vi "SuperAuto.vi"() -> ()   [LabVIEW 2014]
uses:
  Support Files/SuperAutoStates.ctl
  Support Files/Global Data!!!.vi
  <vilib>/addons/control/pid/pid.llb/PID (DBL).vi
  <vilib>/addons/control/pid/NI_PID_pid.lvlib
panel:
  in  "liftEnc":dbl
  in  "elevator":dbl
  in  "autoLift":bool
  in  "rightEnc":dbl
  in  "leftEnc":dbl
  in  "manual?":bool
  in  "ElevatorStateMachine":bool
  in  "gyroAngle":dbl
  in  "Turn":dbl
  in  "Power":dbl
  in  "Extend":bool
  in  "SecondStage":bool
  in  "FirstStage":bool
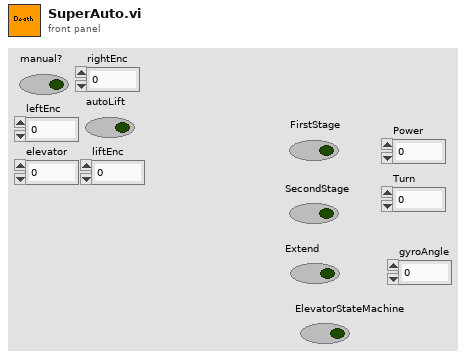
[diagram p1: front panel]
types:
  T1 = typedef "SuperAutoStates.ctl" = enum16{"Grasp RC", "Turn", "Release", "Retract", "2-Stage Process", "Straigten", "Drive Forward", "Done"}
  T2 = cluster{"proportional gain (Kc)":dbl, "integral time (Ti, min)":dbl, "derivative time (Td, min)":dbl}
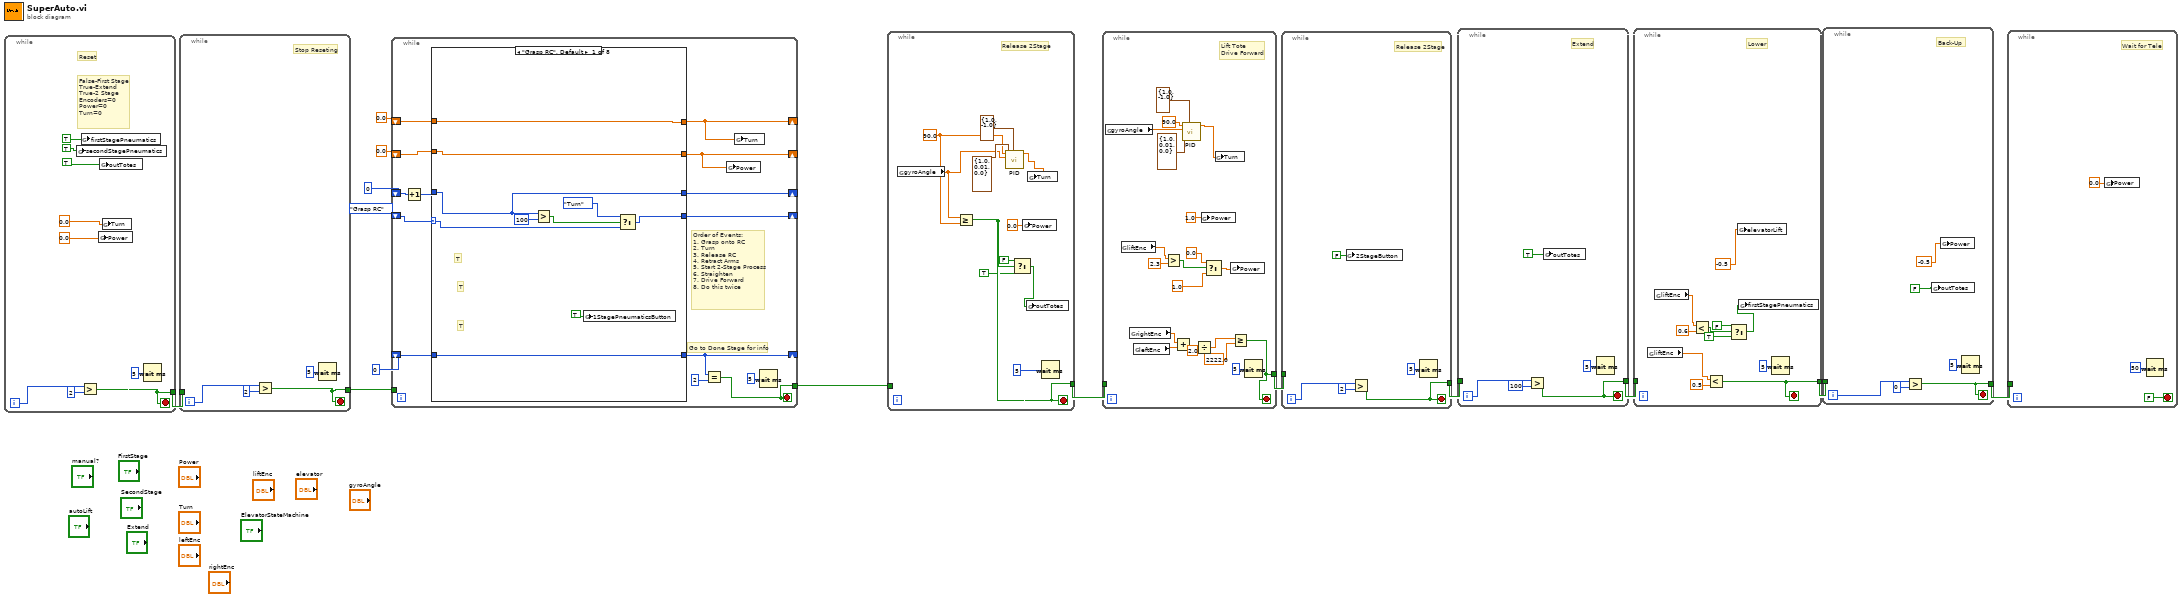
[diagram p0: block diagram]
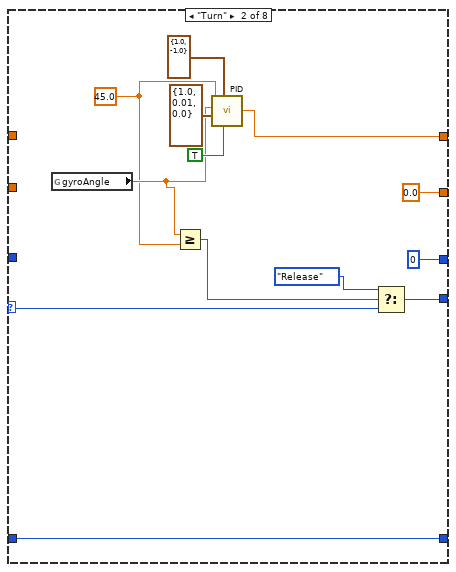
[diagram p2: hidden frame]
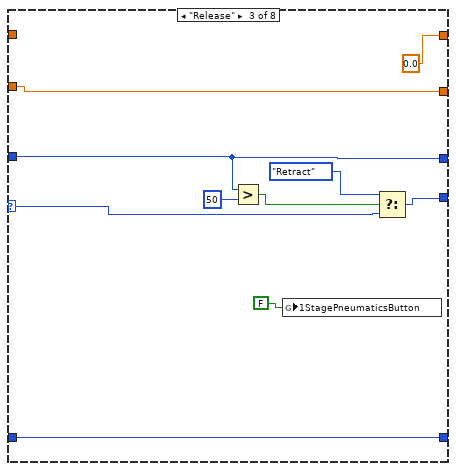
[diagram p3: hidden frame]
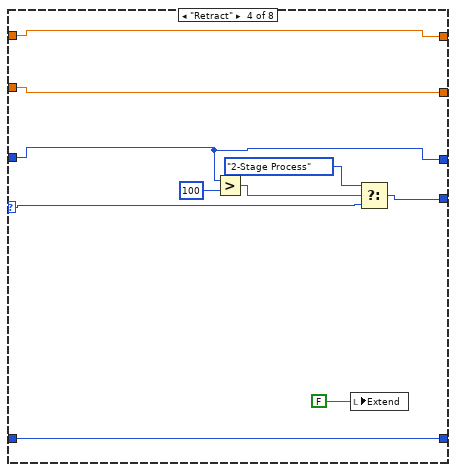
[diagram p4: hidden frame]
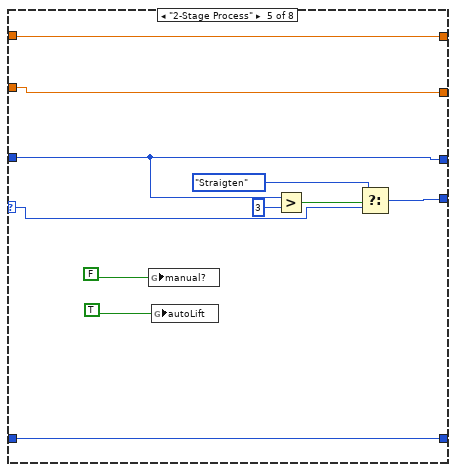
[diagram p5: hidden frame]
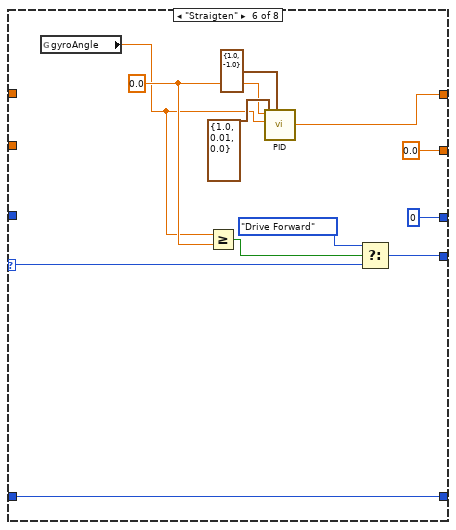
[diagram p6: hidden frame]
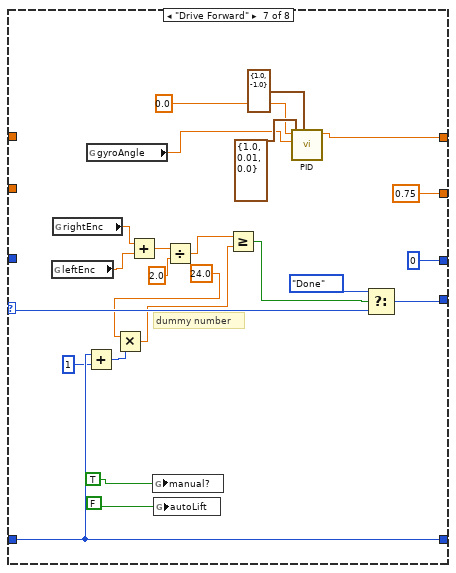
[diagram p7: hidden frame]
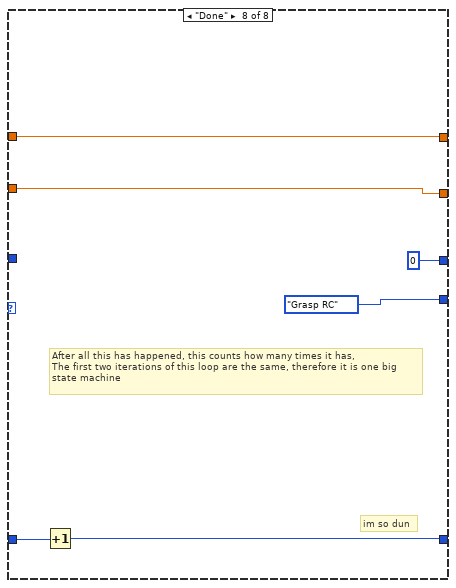
[diagram p8: hidden frame]
diagram:
  n1 = while {
    tunnel: [w20] -> w14
    i -> [w23]
    stop <- w20 stop-if-true
    # "False-First Stage\nTrue-Extend\nTrue-2 Stage\nEncoders=0\nPower=0\nTurn=0"
    # "Reset"
    n2 = global write "Global Data!!!.vi" "secondStagePneumatics"(TRUE) -> ()
    n3 = global write "Global Data!!!.vi" "firstStagePneumatics"(TRUE) -> ()
    n4 = Greater?(x=w23, y=2) -> (0:w20:bool)
    n5 = global write "Global Data!!!.vi" "Power"(0.0) -> ()
    n6 = global write "Global Data!!!.vi" "outTotes"(TRUE) -> ()
    n7 = global write "Global Data!!!.vi" "Turn"(0.0) -> ()
    n8 = Wait (ms)(milliseconds to wait=u32 5) -> ()  [unwired: 1 out]
  }
  n9 = while {
    tunnel: w14 -> [_]
    tunnel: [w24] -> w11
    i -> [w27]
    stop <- w24 stop-if-true
    # "Stop Reseting"
    n10 = Greater?(x=w27, y=2) -> (0:w24:bool)
    n11 = Wait (ms)(milliseconds to wait=u32 5) -> ()  [unwired: 1 out]
  }
  n12 = while {
    shift-right: [w40] -> _
    shift-left: SuperAutoStates."Grasp RC" -> [w41]
    shift-right: [w36] -> _
    shift-left: u32 0 ("milliseconds to wait") -> [w38]
    shift-right: [w29] -> _
    shift-left: 0.0 ("output") -> [w34]
    shift-right: [w28] -> _
    shift-left: 0.0 -> [w35]
    tunnel: w11 -> [_]
    shift-right: [w32] -> _
    shift-left: u32 0 ("milliseconds to wait") -> [w33]
    tunnel: [w30] -> w4
    stop <- w30 stop-if-true
    # "Go to Done Stage for info"
    # "Order of Events: \n1. Grasp onto RC\n2. Turn\n3. Release RC\n4. Retract Arms\n5. Start 2-Stage Process\n6. Straighten\n7. Drive Forward\n8. Do this twice"
    n13 = Increment(x=w38) -> (x+1=w37:u32)
    n14 = case shown="\"Grasp RC\", Default" w41 {
      selector: w41 -> [w51 w62 w69 w77 w92 w102 w126 _]
      tunnel: [w45 w55 0.0 ("output") w82 w89 w99 w120 w133] -> w29
      tunnel: [w44 0.0 w68 w81 w88 0.0 0.75 w132] -> w28
      tunnel: [w50 w63 w66 w75 w94 w103 w127 SuperAutoStates."Grasp RC"] -> w40
      tunnel: w37 -> [w46 _ w70 w76 w87 _ _ _]
      tunnel: [w46 u32 0 w70 w76 w87 u32 0 u32 0 u32 0] -> w36
      tunnel: w35 -> [w44 _ w68 w81 w88 _ _ w132]
      tunnel: w34 -> [w45 _ _ w82 w89 _ _ w133]
      tunnel: [w43 w58 w67 w84 w95 w107 w115 w135] -> w32
      tunnel: w33 -> [w43 w58 w67 w84 w95 w107 w115 w136]
      frame "Grasp RC", Default {
        # "T"
        # "T"
        # "T"
        n15 = Greater?(x=w46, y=u32 100) -> (0:w48:bool)
        n16 = global write "Global Data!!!.vi" "1StagePneumaticsButton"(TRUE) -> ()
        n17 = Select(t=SuperAutoStates."Turn", s=w48, f=w51) -> (s? t:f=w50:T1)
      }
      frame "Turn" {
        w52 = 45.0 ("setpoint")
        n18 = global read "Global Data!!!.vi" "gyroAngle"() -> (w53:dbl)
        n19 = Greater Or Equal?(x=w53, y=w52) -> (x >= y?=w60:bool)
        n20 = call-poly <vilib>:"PID.vi"("reinitialize? (F)"=TRUE, "output range"=cluster{"output high":dbl, "output low":dbl} {"output high"=1.0, "output low"=-1.0}, "PID gains"=T2 {"proportional gain (Kc)"=1.0, "integral time (Ti, min)"=0.01, "derivative time (Td, min)"=0.0}, "process variable"=w53, "setpoint"=w52) -> ("output"=w55:dbl)  [unwired: 5 in, 1 out]
        n21 = Select(t=SuperAutoStates."Release", s=w60, f=w62) -> (s? t:f=w63:T1)
      }
      frame "Release" {
        n22 = Greater?(x=w70, y=u32 50) -> (0:w72:bool)
        n23 = global write "Global Data!!!.vi" "1StagePneumaticsButton"(FALSE) -> ()
        n24 = Select(t=SuperAutoStates."Retract", s=w72, f=w69) -> (s? t:f=w66:T1)
      }
      frame "Retract" {
        n25 = Greater?(x=w76, y=u32 100) -> (0:w79:bool)
        n26 = local write "Extend"(FALSE) -> ()
        n27 = Select(t=SuperAutoStates."2-Stage Process", s=w79, f=w77) -> (s? t:f=w75:T1)
      }
      frame "2-Stage Process" {
        n28 = global write "Global Data!!!.vi" "manual?"(FALSE) -> ()
        n29 = global write "Global Data!!!.vi" "autoLift"(TRUE) -> ()
        n30 = Greater?(x=w87, y=u32 3) -> (0:w93:bool)
        n31 = Select(t=SuperAutoStates."Straigten", s=w93, f=w92) -> (s? t:f=w94:T1)
      }
      frame "Straigten" {
        w105 = 0.0 ("setpoint")
        n32 = global read "Global Data!!!.vi" "gyroAngle"() -> (w96:dbl)
        n33 = Greater Or Equal?(x=w96, y=w105) -> (x >= y?=w100:bool)
        n34 = call-poly <vilib>:"PID.vi"("output range"=cluster{"output high":dbl, "output low":dbl} {"output high"=1.0, "output low"=-1.0}, "PID gains"=T2 {"proportional gain (Kc)"=1.0, "integral time (Ti, min)"=0.01, "derivative time (Td, min)"=0.0}, "process variable"=w96, "setpoint"=w105) -> ("output"=w99:dbl)  [unwired: 6 in, 1 out]
        n35 = Select(t=SuperAutoStates."Drive Forward", s=w100, f=w102) -> (s? t:f=w103:T1)
      }
      frame "Drive Forward" {
        # "dummy number"
        n36 = global read "Global Data!!!.vi" "leftEnc"() -> (w109:dbl)
        n37 = global read "Global Data!!!.vi" "rightEnc"() -> (w108:dbl)
        n38 = Add(x=w115, y=u32 1) -> (x+y=w113:u32)
        n39 = global read "Global Data!!!.vi" "gyroAngle"() -> (w110:dbl)
        n40 = Multiply(x=24.0 ("y"), y=w113) -> (x*y=w111:dbl)
        n41 = Add(x=w108, y=w109) -> (x+y=w130:dbl)
        n42 = global write "Global Data!!!.vi" "manual?"(TRUE) -> ()
        n43 = global write "Global Data!!!.vi" "autoLift"(FALSE) -> ()
        n44 = Divide(x=w130, y=2.0) -> (x/y=w128:dbl)
        n45 = Greater Or Equal?(x=w128, y=w111) -> (x >= y?=w125:bool)
        n46 = call-poly <vilib>:"PID.vi"("output range"=cluster{"output high":dbl, "output low":dbl} {"output high"=1.0, "output low"=-1.0}, "PID gains"=T2 {"proportional gain (Kc)"=1.0, "integral time (Ti, min)"=0.01, "derivative time (Td, min)"=0.0}, "process variable"=w110, "setpoint"=0.0) -> ("output"=w120:dbl)  [unwired: 6 in, 1 out]
        n47 = Select(t=SuperAutoStates."Done", s=w125, f=w126) -> (s? t:f=w127:T1)
      }
      frame "Done" {
        # "After all this has happened, this counts how many times it has,\nThe first two iterations of this loop are the same, therefore it is one big\nstate machine"
        # "im so dun"
        n48 = Increment(x=w136) -> (x+1=w135:u32)
      }
    }
    n49 = Equal?(x=w32, y=u32 2) -> (x = y?=w30:bool)
    n50 = global write "Global Data!!!.vi" "Power"(w28) -> ()
    n51 = global write "Global Data!!!.vi" "Turn"(w29) -> ()
    n52 = Wait (ms)(milliseconds to wait=u32 5) -> ()  [unwired: 1 out]
  }
  n53 = while {
    tunnel: [w143] -> w3
    tunnel: w4 -> [_]
    stop <- w143 stop-if-true
    w144 = 90.0 ("setpoint")
    # "Release 2Stage"
    n54 = global read "Global Data!!!.vi" "gyroAngle"() -> (w140:dbl)
    n55 = Greater Or Equal?(x=w140, y=w144) -> (x >= y?=w143:bool)
    n56 = call-poly <vilib>:"PID.vi"("output range"=cluster{"output high":dbl, "output low":dbl} {"output high"=1.0, "output low"=-1.0}, "PID gains"=T2 {"proportional gain (Kc)"=1.0, "integral time (Ti, min)"=0.01, "derivative time (Td, min)"=0.0}, "process variable"=w140, "setpoint"=w144) -> ("output"=w139:dbl)  [unwired: 6 in, 1 out]
    n57 = Select(t=FALSE, s=w143, f=TRUE ("manual?")) -> (s? t:f=w137:bool)
    n58 = global write "Global Data!!!.vi" "Power"(0.0 ("Power")) -> ()
    n59 = global write "Global Data!!!.vi" "outTotes"(w137) -> ()
    n60 = global write "Global Data!!!.vi" "Turn"(w139) -> ()
    n61 = Wait (ms)(milliseconds to wait=u32 5) -> ()  [unwired: 1 out]
  }
  n62 = while {
    tunnel: [w155] -> w7
    tunnel: w3 -> [_]
    stop <- w155 stop-if-true
    # "Lift Tote\nDrive Forward"
    n63 = global read "Global Data!!!.vi" "gyroAngle"() -> (w153:dbl)
    n64 = global read "Global Data!!!.vi" "liftEnc"() -> (w151:dbl)
    n65 = global read "Global Data!!!.vi" "rightEnc"() -> (w148:dbl)
    n66 = global read "Global Data!!!.vi" "leftEnc"() -> (w149:dbl)
    n67 = Greater?(x=w151, y=2.3) -> (0:w156:bool)
    n68 = Add(x=w148, y=w149) -> (x+y=w162:dbl)
    n69 = call-poly <vilib>:"PID.vi"("output range"=cluster{"output high":dbl, "output low":dbl} {"output high"=1.0, "output low"=-1.0}, "PID gains"=T2 {"proportional gain (Kc)"=1.0, "integral time (Ti, min)"=0.01, "derivative time (Td, min)"=0.0}, "process variable"=w153, "setpoint"=90.0) -> ("output"=w154:dbl)  [unwired: 6 in, 1 out]
    n70 = Divide(x=w162, y=2.0) -> (x/y=w160:dbl)
    n71 = global write "Global Data!!!.vi" "Power"(1.0 ("Power")) -> ()
    n72 = Select(t=0.0, s=w156, f=1.0) -> (s? t:f=w150:dbl)
    n73 = global write "Global Data!!!.vi" "Turn"(w154) -> ()
    n74 = global write "Global Data!!!.vi" "Power"(w150) -> ()
    n75 = Greater Or Equal?(x=w160, y=2222.0) -> (x >= y?=w155:bool)
    n76 = Wait (ms)(milliseconds to wait=u32 5) -> ()  [unwired: 1 out]
  }
  n77 = while {
    tunnel: w7 -> [_]
    tunnel: [w169] -> w5
    i -> [w171]
    stop <- w169 stop-if-true
    # "Release 2Stage"
    n78 = global write "Global Data!!!.vi" "2StageButton"(FALSE ("2StageButton")) -> ()
    n79 = Greater?(x=w171, y=2) -> (0:w169:bool)
    n80 = Wait (ms)(milliseconds to wait=u32 5) -> ()  [unwired: 1 out]
  }
  n81 = while {
    tunnel: [w174] -> w6
    tunnel: w5 -> [_]
    i -> [w176]
    stop <- w174 stop-if-true
    # "Extend"
    n82 = Greater?(x=w176, y=100) -> (0:w174:bool)
    n83 = global write "Global Data!!!.vi" "outTotes"(TRUE ("SecondStage")) -> ()
    n84 = Wait (ms)(milliseconds to wait=u32 5) -> ()  [unwired: 1 out]
  }
  n85 = while {
    tunnel: w6 -> [_]
    tunnel: [w182] -> w2
    stop <- w182 stop-if-true
    # "Lower"
    n86 = global read "Global Data!!!.vi" "liftEnc"() -> (w179:dbl)
    n87 = global read "Global Data!!!.vi" "liftEnc"() -> (w180:dbl)
    n88 = Less?(x=w180, y=0.6) -> (x < y?=w183:bool)
    n89 = Less?(x=w179, y=0.5) -> (x < y?=w182:bool)
    n90 = Select(t=FALSE, s=w183, f=TRUE ("SecondStage")) -> (s? t:f=w178:bool)
    n91 = global write "Global Data!!!.vi" "elevatorLift"(-0.5 ("elevator")) -> ()
    n92 = global write "Global Data!!!.vi" "firstStagePneumatics"(w178) -> ()
    n93 = Wait (ms)(milliseconds to wait=u32 5) -> ()  [unwired: 1 out]
  }
  n94 = while {
    tunnel: w2 -> [_]
    tunnel: [w191] -> w1
    i -> [w193]
    stop <- w191 stop-if-true
    # "Back-Up"
    n95 = Greater?(x=w193, y=0) -> (0:w191:bool)
    n96 = global write "Global Data!!!.vi" "outTotes"(FALSE ("SecondStage")) -> ()
    n97 = global write "Global Data!!!.vi" "Power"(-0.5 ("elevator")) -> ()
    n98 = Wait (ms)(milliseconds to wait=u32 5) -> ()  [unwired: 1 out]
  }
  n99 = while {
    tunnel: w1 -> [_]
    stop <- FALSE stop-if-true
    # "Wait for Tele"
    n100 = global write "Global Data!!!.vi" "Power"(0.0 ("Power")) -> ()
    n101 = Wait (ms)(milliseconds to wait=u32 50) -> ()  [unwired: 1 out]
  }
